vi "initialise data processor variables.vi"(11 "dataProcessor in":T1) -> (0 "error out":errorcluster, 3 "dataProcessor out":T1)   [LabVIEW 2018]
uses:
  type defs/data processor data.ctl
  type defs/channelLimitControl.ctl
  type defs/limitActions.ctl
  Chris VIs/data channels/parent class/Data Channel.lvclass
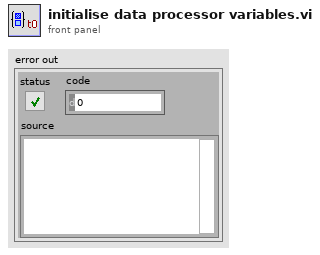
[diagram p1: front panel]
types:
  T1 = typedef "data processor data.ctl" = cluster{"params":cluster{"controlFeedback":cluster{"butterflyValue":u16, "ballValue":u16, "massflow":u16, "pressureRatio":u16, "compSpeed":u16}, "DAQrate":enum16{"50 kHz", "25 kHz", "16.6 kHz", "12.5 kHz", "10 kHz", "8.33 kHz", "7.14 kHz", "6.25 kHz", "5.55 kHz", "5 kHz"}, "safetyChannels":cluster{"oilP":u16, "airP":u16, "water":u16, "channelLimit":T2[]}, "channelConfigPath":path}, "vars":cluster{"controlFeedback":cluster{"butterflyValue":u16, "ballValue":u16, "massflow":u16, "pressureRatio":u16, "compSpeed":u16}, "activeChannelNames":string[], "activeChannelUnits":string[], "offset trigger":bool, "offsets":dbl[], "activeChannelLimitIndex":u16[], "liveData":bool}}
  T2 = typedef "channelLimitControl.ctl" = cluster{"channelID":u16, "Enabled":bool, "warnValue":dbl, "limitValue":dbl, "Invert":bool, "limitAction":T3}
  T3 = typedef "limitActions.ctl" = enum16{"stop", "shutdown", "ignore"}
  T4 = typedef "channelControl.ctl" = cluster{"index":u16, "active":bool, "channelType":T5, "module":u16, "terminal":u16, "channelName":string, "scalingMethod":T6, "scalingParameters":dbl[], "scaledUnits":string, "tempOffset":dbl}
  T5 = typedef "channelScalingTypes.ctl" = enum16{"calculation", "measurement", "scanivalve", "output", "digital"}
  T6 = typedef "scalingMethods.ctl" = enum16{"none", "linear", "thermocouple", "polynomial", "encoder", "RTD"}
  T7 = typedef "Data Channel.lvclass/basic channel details.ctl" = cluster{"index":u16, "Active":bool, "channel name":string, "units":string, "module":string, "port":string, "liveOffset":dbl, "precision":u8, "channelType":T8, "fifoIndex":u16, "dataSource":T9, "acquireIndex":u16}
  T8 = typedef "Data Channel.lvclass/channel type.ctl" = enum16{"acquisition", "output", "other"}
  T9 = typedef "Data Channel.lvclass/dataSource.ctl" = enum16{"Not available", "FIFO", "Scanivalve", "Remote", "Calculated"}
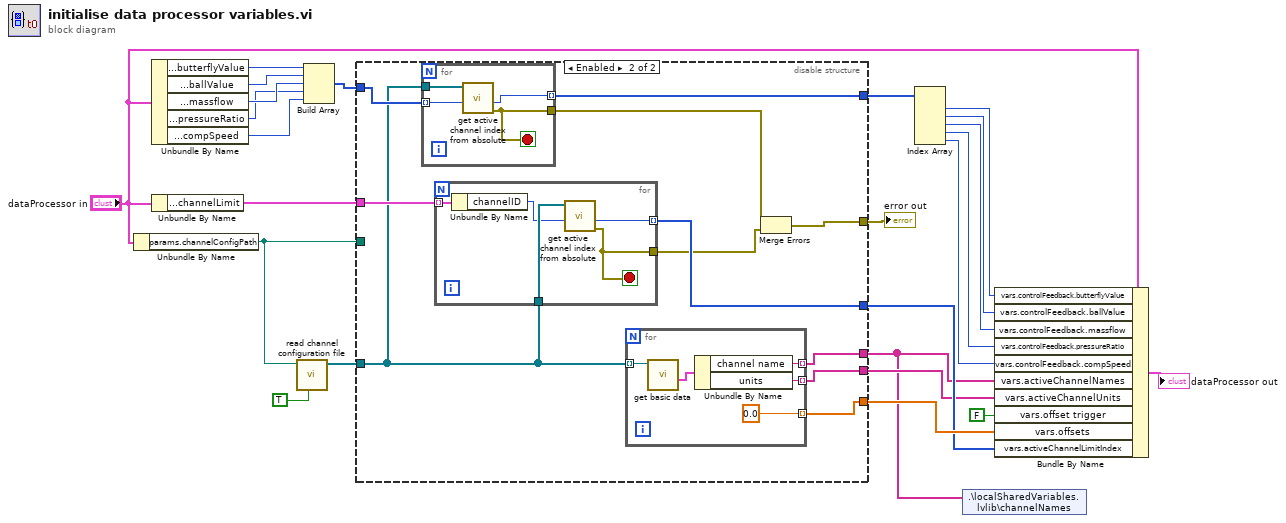
[diagram p0: block diagram]
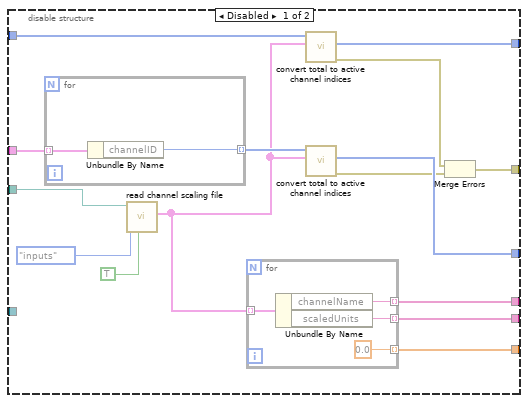
[diagram p2: hidden frame]
diagram:
  n1 = Unbundle By Name("dataProcessor in") -> ("params.channelConfigPath"=w10:path)
  n2 = Unbundle By Name("dataProcessor in") -> ("params.controlFeedback.butterflyValue"=w23:u16, "params.controlFeedback.ballValue"=w22:u16, "params.controlFeedback.massflow"=w7:u16, "params.controlFeedback.pressureRatio"=w6:u16, "params.controlFeedback.compSpeed"=w5:u16)
  n3 = Unbundle By Name("dataProcessor in") -> ("params.safetyChannels.channelLimit"=w14:T2[])
  n4 = call "read channel configuration file.vi"("Hide inactive (F)"=TRUE, "config file"=w10) -> ("channelsArray"=w8:refnum<class "Data Channel.lvclass">[])  [unwired: 7 in, 2 out]
  n5 = Build Array(w23, w22, w7, w6, w5) -> (w21:u16[])
  n6 = disable-structure shown="Enabled" {
    disable-tunnel: w21 -> [w37 w53]
    disable-tunnel: [w36 w52] -> w20
    disable-tunnel: [w35 w54] -> w16
    disable-tunnel: w14 -> [w32 w50]
    disable-tunnel: [w31 w48] -> w13
    disable-tunnel: [w28 w47] -> w12
    disable-tunnel: [w27 w56] -> w1
    disable-tunnel: [w26 w55] -> w11
    disable-tunnel: w10 -> [w25 _]
    disable-tunnel: w8 -> [_ w49]
    frame Disabled {
      n7 = for {
        tunnel: [w44] -> w34 mode=indexing
        tunnel: w32 -> [w45] mode=indexing
        n8 = Unbundle By Name(w45) -> ("channelID"=w44:u16)
      }
      n9 = call "read channel scaling file.vi"("suppress inactive? (F)"=TRUE, "mode (all)"=enum16{"all", "inputs", "outputs", "digital"}."inputs", "file path"=w25) -> ("channelConfig"=w33:T4[])  [unwired: 4 in, 4 out]
      n10 = for {
        tunnel: w33 -> [w43] mode=indexing
        tunnel: [w42] -> w27 mode=indexing
        tunnel: [w41] -> w26 mode=indexing
        tunnel: [0.0] -> w35 mode=indexing
        n11 = Unbundle By Name(w43) -> ("channelName"=w42:string, "scaledUnits"=w41:string)
      }
      n12 = call "convert total to active channel indices.vi"("channelConfig"=w33, "AbsoluteChannelIndices"=w37) -> ("error out"=w30:errorcluster, "activeChannelIndices"=w36:u16[])  [unwired: 8 in]
      n13 = call "convert total to active channel indices.vi"("channelConfig"=w33, "AbsoluteChannelIndices"=w34) -> ("error out"=w29:errorcluster, "activeChannelIndices"=w31:u16[])  [unwired: 8 in]
      n14 = Merge Errors(w30, w29) -> (w28:errorcluster)
    }
    frame Enabled {
      n15 = for {
        tunnel: w49 -> [w65]
        tunnel: w53 -> [w64] mode=indexing
        tunnel: [w63] -> w52 mode=indexing
        tunnel: [w62] -> w51
        stop <- w62 stop-if-true
        n16 = call "get active channel index from absolute.vi"("absoluteIndex"=w64, "channels"=w65) -> ("error"=w62:errorcluster, "activeIndex"=w63:u16)  [unwired: 8 in]
      }
      n17 = for {
        tunnel: w50 -> [w61] mode=indexing
        tunnel: w49 -> [w60]
        tunnel: [w58] -> w48 mode=indexing
        tunnel: [w57] -> w46
        stop <- w57 stop-if-true
        n18 = Unbundle By Name(w61) -> ("channelID"=w59:u16)
        n19 = call "get active channel index from absolute.vi"("absoluteIndex"=w59, "channels"=w60) -> ("error"=w57:errorcluster, "activeIndex"=w58:u16)  [unwired: 8 in]
      }
      n20 = for {
        tunnel: [w69] -> w56 mode=indexing
        tunnel: [w68] -> w55 mode=indexing
        tunnel: [0.0] -> w54 mode=indexing
        tunnel: w49 -> [w66] mode=indexing
        n21 = call "get basic data.vi"("Data Channel in"=w66) -> ("details"=w70:T7)  [unwired: 9 in, 1 out]
        n22 = Unbundle By Name(w70) -> ("channel name"=w69:string, "units"=w68:string)
      }
      n23 = Merge Errors(w51, w46) -> (w47:errorcluster)
    }
  }
  "error out" <- w12
  n24 = Index Array(array=w20) -> (element #1=w19:u16, element #2=w18:u16, element #3=w4:u16, element #4=w3:u16, element #5=w2:u16)  [unwired: 5 in]
  n25 = shared-variable ".\\localSharedVariables.lvlib\\channelNames"(w1) -> ()  [unwired: 1 in, 1 out]
  n26 = Bundle By Name(cluster="dataProcessor in", "vars.controlFeedback.butterflyValue"=w19, "vars.controlFeedback.ballValue"=w18, "vars.controlFeedback.massflow"=w4, "vars.controlFeedback.pressureRatio"=w3, "vars.controlFeedback.compSpeed"=w2, "vars.activeChannelNames"=w1, "vars.activeChannelUnits"=w11, "vars.offset trigger"=FALSE, "vars.offsets"=w16, "vars.activeChannelLimitIndex"=w13) -> (→"dataProcessor out":T1)
